vi "Multiply Rational Polynomials (DBL).vi"(4 "threshold type":T1 items=["Absolute Value", "Relative Value"], 6 "threshold":dbl, 8 "Denominator 2":dbl[](array[numeric]) format="%#.2g", 9 "Numerator 2":dbl[](array[numeric]) format="%#.2p", 10 "Denominator 1":dbl[](array[numeric]) format="%#.2g", 11 "Numerator 1":dbl[](array[numeric]) format="%#.2p") -> (0 "error":i32, 2 "Denominator Out":dbl[](array[numeric]) format="%#.2g", 3 "Numerator Out":dbl[](array[numeric]) format="%#.2g")   [LabVIEW 2010, in "NI_AALPro.lvlib"]
doc: "Multiplies rational polynomial G1 by rational polynomial G2. The data types you wire to the <B>Numerator 1</B>, <B>Denominator 1</B>, <B>Numerator 2</B>, and <B>Denominator 2</B> inputs determine the polymorphic instance to use."
uses:
  NI_AALPro.lvlib
  Remove Zero Threshold Type.ctl
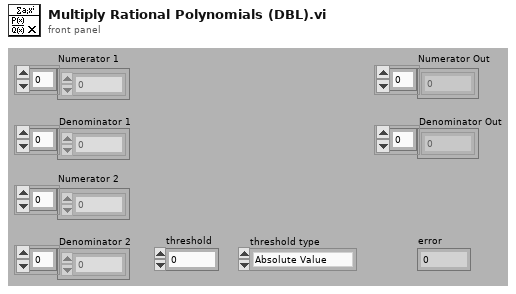
[diagram p1: front panel]
types:
  T1 = typedef "NI_AALPro.lvlib/Remove Zero Threshold Type.ctl" = u16
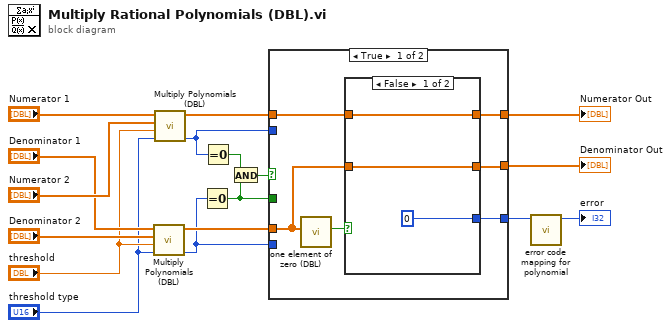
[diagram p0: block diagram]
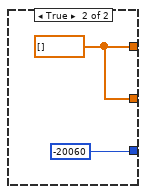
[diagram p2: hidden frame]
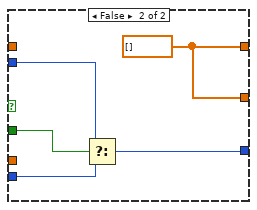
[diagram p3: hidden frame]
diagram:
  n1 = call "Multiply Polynomials (DBL).vi"("threshold type"="threshold type", "threshold"="threshold", "Q(x)"="Denominator 2", "P(x)"="Denominator 1") -> ("error"=w6:i32, "P(x)*Q(x)"=w10:dbl[])  [unwired: 6 in]
  n2 = call "Multiply Polynomials (DBL).vi"("threshold type"="threshold type", "threshold"="threshold", "Q(x)"="Numerator 2", "P(x)"="Numerator 1") -> ("error"=w7:i32, "P(x)*Q(x)"=w15:dbl[])  [unwired: 6 in]
  n3 = Equal To 0?(x=w6) -> (x = 0?=w3:bool)
  n4 = Equal To 0?(x=w7) -> (x = 0?=w5:bool)
  n5 = And(x=w5, y=w3) -> (x .and. y?=w4:bool)
  n6 = case shown="True" w4 {
    tunnel: w15 -> [w21 _]
    tunnel: [w20 w33] -> w14
    tunnel: [w18 w33] -> w13
    tunnel: w10 -> [w19 _]
    tunnel: [w23 w30] -> w9
    tunnel: w7 -> [_ w32]
    tunnel: w6 -> [_ w31]
    tunnel: w3 -> [_ w29]
    frame True {
      n7 = call "one element of zero (DBL).vi"("Array in"=w19) -> ("equal [0]?"=w22:bool)  [unwired: 10 in]
      n8 = case shown="False" w22 {
        tunnel: [0 -20060 ("divide by zero")] -> w23
        tunnel: w21 -> [w25 _]
        tunnel: [w25 w28] -> w20
        tunnel: w19 -> [w24 _]
        tunnel: [w24 w28] -> w18
        frame False {
        }
        frame True {
          w28 = dbl[] [] ("BDL")
        }
      }
    }
    frame False {
      w33 = dbl[] [] ("BDL")
      n9 = Select(t=w32, s=w29, f=w31) -> (s? t:f=w30:i32)
    }
  }
  "Numerator Out" <- w14
  "Denominator Out" <- w13
  n10 = call "error code mapping for polynomial.vi"("error in"=w9) -> ("error out"=→"error":i32)  [unwired: 10 in]
